vi "OP400ZP_OCVmax.vi"() -> ()   [LabVIEW 2020]
panel:
  out "OCVmax":dbl
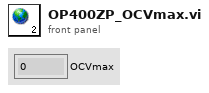
[diagram p1: front panel]
diagram:
